vi "loadSettings.vi"(8 "error in (no error)":errorcluster, 11 "TaskRef in":refnum<vi>) -> (0 "error out":errorcluster, 3 "TaskRef out":refnum<vi>)   [LabVIEW 2015, in "pdbm_tasks.lvlib"]
doc: "reload setting file and initialize value to controls on VI. Default value will be assigned to control if setting file is not found.\n<b>Note</b>: setting file is placed in Config folder in application root folder and named as <b><VI_name>_setting.xml<b/>"
uses:
  pdbm_tasks.lvlib
  <vilib>/NI/GXML/Compatibility/gxml_QuickParser.vi
  <vilib>/NI/GXML/Read XML from File.vi
  <vilib>/NI/GXML/_subVIs/GXML Quick Parser/Quick Parser.vi
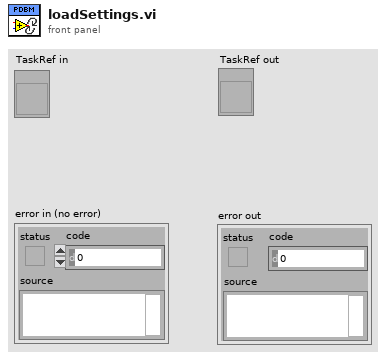
[diagram p1: front panel]
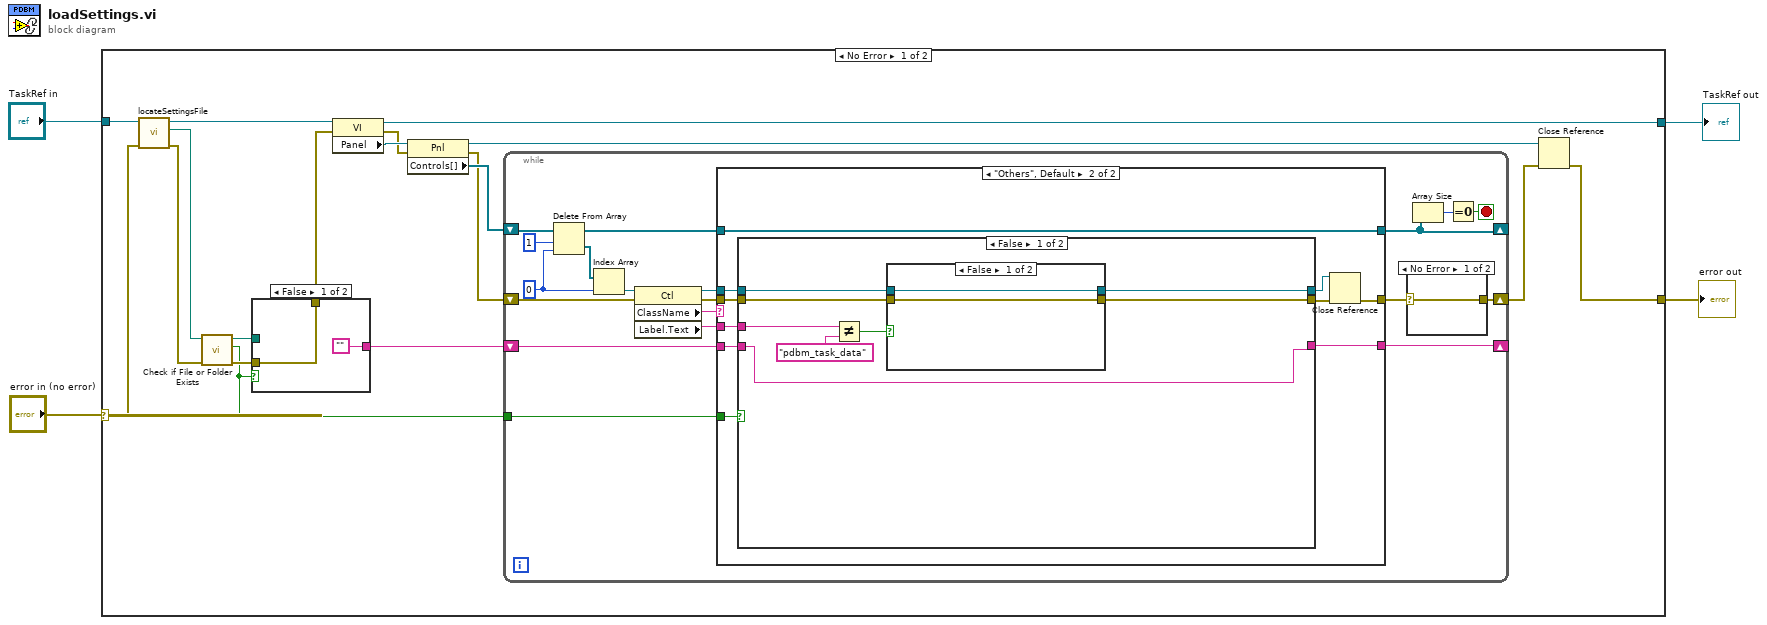
[diagram p0: block diagram]
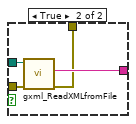
[diagram p2: hidden frame]
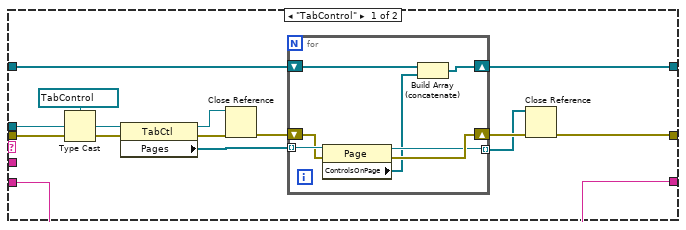
[diagram p4: hidden frame]
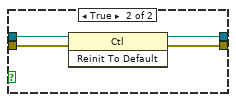
[diagram p5: hidden frame]
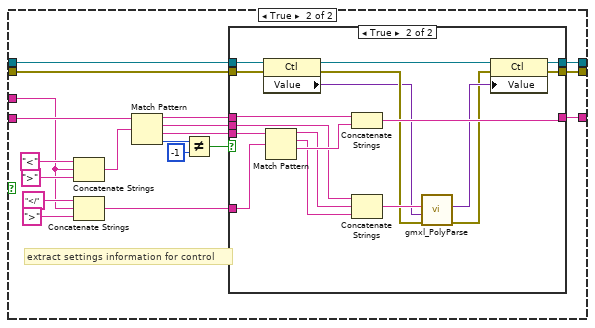
[diagram p6: hidden frame]
diagram:
  n1 = case shown="No Error" "error in (no error)" {
    selector: "error in (no error)" -> [w18 w134]
    tunnel: "TaskRef in" -> [w16 w135]
    tunnel: [w20 w135] -> w2
    tunnel: [w19 w134] -> w1
    frame No Error {
      n2 = call "locateSettingsFile.vi"("error in (no error)"=w18, "VI Refnum in"=w16) -> ("error out"=w17:errorcluster, "path"=w15:path, "VI Refnum out"=w14:refnum<vi>)  [unwired: 7 in]
      n3 = call <vilib>:"Check if File or Folder Exists.vi"("error in (no error)"=w17, "path"=w15) -> ("error out"=w21:errorcluster, "file or folder exists?"=w5:bool, "dup path"=w22:path)  [unwired: 7 in]
      n4 = case shown="False" w5 {
        tunnel: w22 -> [_ w28]
        tunnel: w21 -> [w24 w27]
        tunnel: ["" w26] -> w9
        tunnel: [w24 w25] -> w8
        frame False {
        }
        frame True {
          n5 = call <vilib>:"gxml_ReadXMLfromFile.vi"("error in"=w27, "XML File Path"=w28) -> ("error out"=w25:errorcluster, "XML String Out"=w26:string)  [unwired: 7 in, 1 out]
        }
      }
      n6 = property class="VI"(reference=w14, error in=w8) -> (reference out=w20:refnum<vi>, error out=w12:errorcluster, "Panel"=w13:refnum<vi>)
      n7 = property class="Pnl"(reference=w13, error in=w12) -> (reference out=w7:refnum<vi>, error out=w10:errorcluster, "Controls[]"=w11:refnum<vi>[])
      n8 = while {
        shift-right: [w30] -> w6
        shift-left: w10 -> [w47]
        shift-right: [w45] -> _
        shift-left: w9 -> [w46]
        shift-right: [w34] -> _
        shift-left: w11 -> [w42]
        tunnel: w5 -> [w29]
        stop <- w33 stop-if-true
        w40 = 0 ("index")
        n9 = Delete From Array(array=w42, length=1, index=w40) -> (deleted portion=w38:refnum<vi>[], array with subset deleted=w35:refnum<vi>[])
        n10 = Index Array(array=w38, index=w40) -> (element=w39:refnum<vi>)
        n11 = property class="Ctl"(reference=w39, error in=w47) -> (reference out=w44:refnum<vi>, error out=w43:errorcluster, "ClassName"=w36:string, "Label.Text"=w37:string)
        n12 = case shown="\"Others\", Default" w36 {
          tunnel: w46 -> [w49 w79]
          tunnel: [w49 w78] -> w45
          tunnel: w44 -> [w62 w74]
          tunnel: w43 -> [w59 w77]
          tunnel: [w51 w70] -> w31
          tunnel: w37 -> [_ w76]
          tunnel: w35 -> [w54 w75]
          tunnel: [w53 w75] -> w34
          tunnel: w29 -> [_ w73]
          frame "TabControl" {
            n13 = Type Cast(type=refnum<vi> refnum ("Tab Control 2"), x=w62) -> (*(type *) &x=w60:refnum<vi>)
            n14 = property class="TabCtl"(reference=w60, error in=w59) -> (reference out=w57:refnum<vi>, error out=w58:errorcluster, "Pages"=w56:refnum<vi>[])
            n15 = Close Reference(reference=w57, error in (no error)=w58) -> (error out=w55:errorcluster)
            n16 = for {
              tunnel: w56 -> [w69] mode=indexing
              shift-right: [w67] -> w52
              shift-left: w55 -> [w68]
              tunnel: [w66] -> w50 mode=indexing
              shift-right: [w63] -> w53
              shift-left: w54 -> [w65]
              n17 = property class="Page"(reference=w69, error in=w68) -> (reference out=w66:refnum<vi>, error out=w67:errorcluster, "ControlsOnPage"=w64:refnum<vi>[])
              n18 = Build Array (concatenate)(w65, w64) -> (w63:refnum<vi>[])
            }
            n19 = Close Reference(reference=w50, error in (no error)=w52) -> (error out=w51:errorcluster)
          }
          frame "Others", Default {
            n20 = case shown="False" w73 {
              tunnel: w79 -> [w80 w112]
              tunnel: [w80 w99] -> w78
              tunnel: w77 -> [w82 w98]
              tunnel: w76 -> [w87 w97]
              tunnel: [w81 w95] -> w72
              tunnel: w74 -> [w84 w96]
              tunnel: [w83 w94] -> w71
              frame False {
                n21 = Not Equal?(x=w87, y="pdbm_task_data") -> (x != y?=w85:bool)
                n22 = case shown="False" w85 {
                  tunnel: [w89 w91] -> w83
                  tunnel: w84 -> [w89 w93]
                  tunnel: w82 -> [w88 w92]
                  tunnel: [w88 w90] -> w81
                  frame False {
                  }
                  frame True {
                    n23 = invoke class="Ctl" method="Reinit To Default"(reference=w93, error in=w92) -> (reference out=w91:refnum<vi>, error out=w90:errorcluster)  [unwired: 1 in, 1 out]
                  }
                }
              }
              frame True {
                # "extract settings information for control"
                n24 = Concatenate Strings("<" ("string"), w97, ">" ("string")) -> (w109:string)
                n25 = Concatenate Strings("</" ("string"), w97, ">" ("string")) -> (w102:string)
                n26 = Match Pattern(string=w112, regular expression=w109) -> (before substring=w101:string, match substring=w100:string, after substring=w104:string, offset past match=w106:i32)  [unwired: 1 in]
                n27 = Not Equal?(x=w106, y=-1) -> (x != y?=w103:bool)
                n28 = case shown="True" w103 {
                  tunnel: w104 -> [_ w133]
                  tunnel: w102 -> [_ w132]
                  tunnel: w101 -> [w115 w130]
                  tunnel: [w115 w131] -> w99
                  tunnel: w100 -> [_ w128]
                  tunnel: w96 -> [w113 w125]
                  tunnel: w98 -> [w114 w124]
                  tunnel: [w113 w117] -> w94
                  tunnel: [w114 w116] -> w95
                  frame False {
                  }
                  frame True {
                    n29 = property class="Ctl"(reference=w125, error in=w124) -> (reference out=w123:refnum<vi>, error out=w121:errorcluster, "Value"=w120:variant)
                    n30 = Match Pattern(string=w133, regular expression=w132) -> (before substring=w127:string, match substring=w126:string, after substring=w129:string)  [unwired: 1 in, 1 out]
                    n31 = Concatenate Strings(w130, w129) -> (w131:string)
                    n32 = Concatenate Strings(w128, w127, w126) -> (w122:string)
                    n33 = call-poly <vilib>:"gmxl_PolyParse.vi"("error in (no error)"=w121, "TypeDesc"=w120, "XML File String"=w122) -> ("error out"=w118:errorcluster, "Parsed Data"=w119:variant)  [unwired: 7 in]
                    n34 = property class="Ctl"(reference=w123, error in=w118, "Value"=w119) -> (reference out=w117:refnum<vi>, error out=w116:errorcluster)
                  }
                }
              }
            }
            n35 = Close Reference(reference=w71, error in (no error)=w72) -> (error out=w70:errorcluster)
          }
        }
        n36 = case shown="No Error" w31 {
          selector: w31 -> [w48 _]
          tunnel: [w48 _] -> w30
          frame No Error {
          }
          frame Error {
          }
        }
        n37 = Array Size(array=w34) -> (size(s)=w32:i32)
        n38 = Equal To 0?(x=w32) -> (x = 0?=w33:bool)
      }
      n39 = Close Reference(reference=w7, error in (no error)=w6) -> (error out=w19:errorcluster)
    }
    frame Error {
    }
  }
  "error out" <- w1
  "TaskRef out" <- w2
